vi "Order Plot Axis.vi"(8 "Order":enum16{"ascending", "descending"}(ring), 10 "Plot Values":dbl[](array[numeric]), 11 "Plot Axis":dbl[](array[numeric])) -> (2 "Ordered Axis Plot Values":dbl[](array[numeric]), 3 "Ordered Plot Axis":dbl[](array[numeric]))   [LabVIEW 2019]
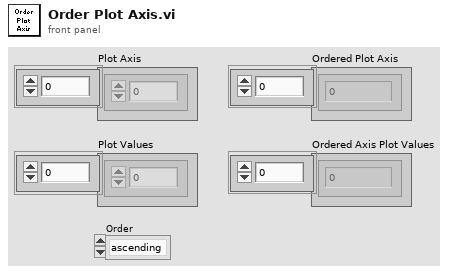
[diagram p1: front panel]
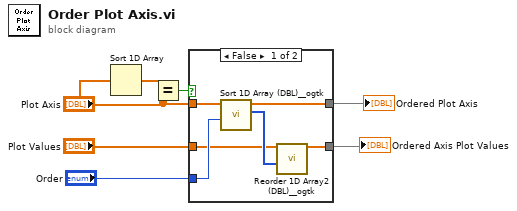
[diagram p0: block diagram]
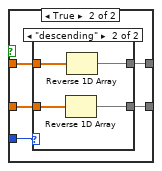
[diagram p2: hidden frame]
diagram:
  n1 = Sort 1D Array(array="Plot Axis") -> (sorted array=w7:dbl[])
  n2 = Equal?(x=w7, y="Plot Axis") -> (x = y?=w6:bool)
  n3 = case shown="False" w6 {
    tunnel: "Plot Values" -> [w9 w16]
    tunnel: [w11 w15] -> w3
    tunnel: "Plot Axis" -> [w13 w17]
    tunnel: [w8 w14] -> w2
    tunnel: "Order" -> [w12 w18]
    frame False {
      n4 = call <userlib>:"Sort 1D Array (DBL)__ogtk.vi"("Order"=w12, "Array in"=w13) -> ("Sorted Pointers"=w10:i32[], "Sorted Array out"=w11:dbl[])  [unwired: 8 in]
      n5 = call <userlib>:"Reorder 1D Array2 (DBL)__ogtk.vi"("indices"=w10, "array"=w9) -> ("reordered array"=w8:dbl[])  [unwired: 9 in]
    }
    frame True {
      n6 = case shown="\"descending\"" w18 {
        tunnel: w17 -> [w20 w24]
        tunnel: w16 -> [w19 w22]
        tunnel: [w20 w23] -> w15
        tunnel: [w19 w21] -> w14
        frame "ascending", Default {
        }
        frame "descending" {
          n7 = Reverse 1D Array(array=w22) -> (reversed array=w21:dbl[])
          n8 = Reverse 1D Array(array=w24) -> (reversed array=w23:dbl[])
        }
      }
    }
  }
  "Ordered Plot Axis" <- w3
  "Ordered Axis Plot Values" <- w2
